vi "Read hasChild_.vi"(8 "error in (no error)":errorcluster, 11 "Snake in":refnum<class "Snake.lvclass">) -> (0 "error out":errorcluster, 2 "hasChild?":bool, 3 "Snake out":refnum<class "Snake.lvclass">)   [LabVIEW 2019, in "Snake.lvclass"]
uses:
  Snake.lvclass
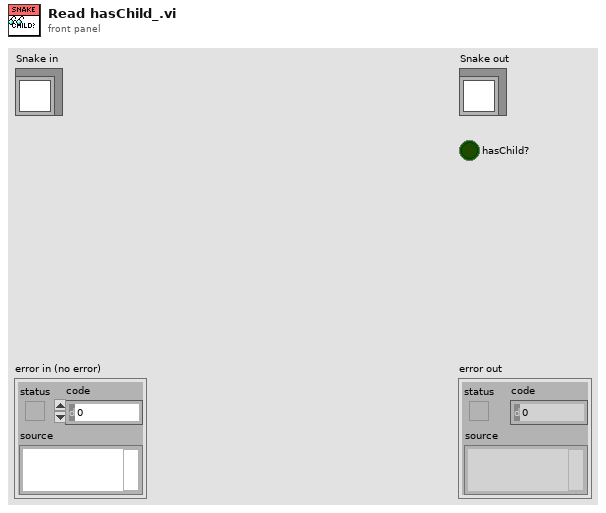
[diagram p1: front panel]
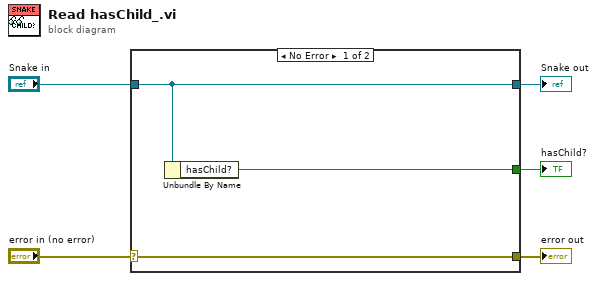
[diagram p0: block diagram]
diagram:
  n1 = case shown="No Error" "error in (no error)" {
    selector: "error in (no error)" -> [w8 w9]
    tunnel: [w8 w9] -> w4
    tunnel: [w7 w10] -> w2
    tunnel: "Snake in" -> [w7 w10]
    tunnel: [w6 _] -> w1
    frame No Error {
      n2 = Unbundle By Name(w7) -> ("hasChild?"=w6:bool)
    }
    frame Error {
    }
  }
  "error out" <- w4
  "Snake out" <- w2
  "hasChild?" <- w1
